vi "RSZVB Get Alternate Sweep Mode.vi"(8 "error in (no error)":errorcluster {"code" format="%.0x"}, 10 "Channel (1)":i32=1, 11 "VISA session":refnum<visa-resource-name>) -> (0 "error out":errorcluster {"code" format="%.0x"}, 2 "Alternate Sweep Mode":i32, 3 "dup VISA session":refnum<visa-resource-name>)   [LabVIEW 2011]
doc: "This VI returns the state of the alternate sweep mode.\n\nNote(s):\n\n(1) This VI is available only on R&S ZVA instrument.\n\nRemote-control command(s):\n[SENSe<Ch>:]COUPle?"
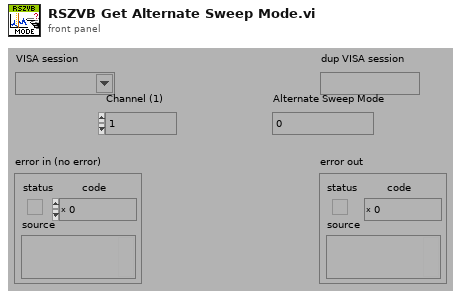
[diagram p1: front panel]
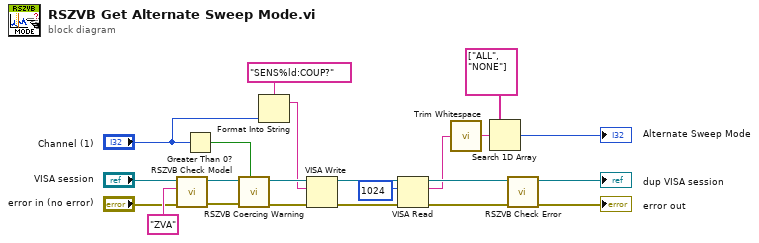
[diagram p0: block diagram]
diagram:
  n1 = call "RSZVB Check Model.vi"("error in (no error)"="error in (no error)", "Model"="ZVA" ("Options"), "VISA session"="VISA session") -> ("error out"=w3:errorcluster, "dup VISA session"=w4:refnum<visa-resource-name>)  [unwired: 7 in]
  n2 = Greater Than 0?(x="Channel (1)") -> (x > 0?=w13:bool)
  n3 = call "RSZVB Coercing Warning.vi"("In Range?"=w13, "error in (no error)"=w3, "VISA session"=w4) -> ("error out"=w20:errorcluster, "dup VISA session"=w21:refnum<visa-resource-name>)  [unwired: 7 in]
  n4 = Format Into String(format string="SENS%ld:COUP?", "Channel (1)") -> (resulting string=w19:string)  [unwired: 2 in, 1 out]
  n5 = VISA Write(VISA resource name=w21, write buffer=w19, error in (no error)=w20) -> (VISA resource name out=w16:refnum<visa-resource-name>, error out=w18:errorcluster)  [unwired: 1 out]
  n6 = VISA Read(VISA resource name=w16, byte count=u32 1024 ("byte count (0)"), error in (no error)=w18) -> (VISA resource name out=w15:refnum<visa-resource-name>, read buffer=w10:string, error out=w14:errorcluster)  [unwired: 1 out]
  n7 = call <vilib>:"Trim Whitespace.vi"("string"=w10) -> ("trimmed string"=w11:string)  [unwired: 1 in]
  n8 = Search 1D Array(1D array=string[] ["ALL", "NONE"] ("array 2"), element=w11) -> (index of element=→"Alternate Sweep Mode":i32)  [unwired: 1 in]
  n9 = call "RSZVB Check Error.vi"("error in (no error)"=w14, "VISA session"=w15) -> ("error out"=→"error out":errorcluster, "dup VISA session"=→"dup VISA session":refnum<visa-resource-name>)  [unwired: 8 in]
